vi "EEGstatus.vi"() -> (3 "Is minima found?":bool)   [LabVIEW 2013]
panel:
  out "sign bits:\n191 for -1\n 63   for  1":u8
  in  "Stop":bool
  out "binary data in ASCII":string
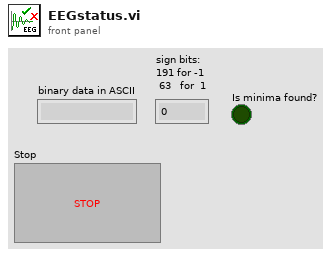
[diagram p1: front panel]
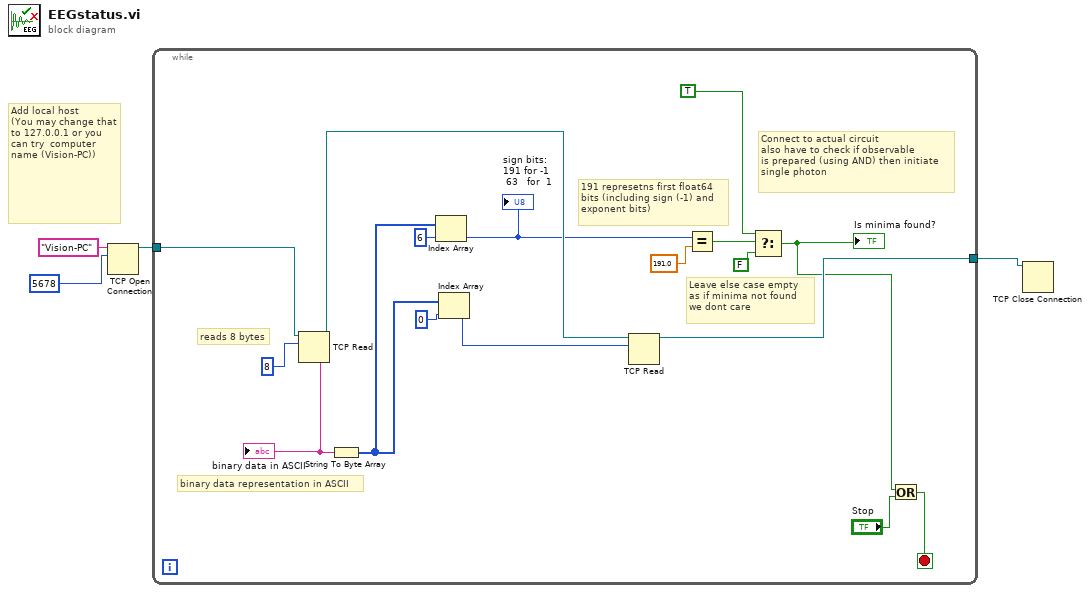
[diagram p0: block diagram]
diagram:
  # "Add local host\n(You may change that to 127.0.0.1 or you can try  computer name (Vision-PC))"
  n1 = TCP Open Connection(address="Vision-PC", remote port or service name=u16 5678) -> (connection ID=w1:refnum<k5>)  [unwired: 3 in, 1 out]
  n2 = while {
    tunnel: [w19] -> w4
    tunnel: w1 -> [w18]
    stop <- w6 stop-if-true
    # "binary data representation in ASCII"
    # "reads 8 bytes"
    # "Leave else case empty\nas if minima not found \nwe dont care"
    # "Connect to actual circuit\nalso have to check if observable \nis prepared (using AND) then initiate\nsingle photon"
    # "191 represetns first float64\nbits (including sign (-1) and\nexponent bits)"
    n3 = TCP Read(connection ID=w18, bytes to read=8) -> (connection ID out=w21:refnum<k5>, data out=w17:string)  [unwired: 3 in, 1 out]
    "binary data in ASCII" <- w17
    n4 = String To Byte Array(string=w17) -> (unsigned byte array=w13:u8[])
    n5 = Index Array(array=w13, index=6) -> (element=w11:u8)
    "sign bits:\n191 for -1\n 63   for  1" <- w11
    n6 = Index Array(array=w13, index=0) -> (element=w16:u8)
    n7 = TCP Read(connection ID=w21, bytes to read=w16) -> (connection ID out=w19:refnum<k5>)  [unwired: 3 in, 2 out]
    n8 = Equal?(x=w11, y=191.0) -> (x = y?=w10:bool)
    n9 = Select(t=TRUE, s=w10, f=FALSE) -> (s? t:f=w5:bool)
    "Is minima found?" <- w5
    n10 = Or(x=w5, y="Stop") -> (x .or. y?=w6:bool)
  }
  n11 = TCP Close Connection(connection ID=w4) -> ()  [unwired: 2 in, 2 out]
